vi "DecodeStreamResponse.vi"(0 "Buffer":string) -> (18 "ChecksumVerified":bool, 19 "Flags":u32, 20 "Gyroscope Full Scale Range":u32, 21 "Accelerometer Full Scale Range":u32, 22 "Output Rate":u32, 23 "Calibrated Yaw Offset":dbl, 24 "Calibrated Quaternion W Offset":u32, 25 "Calibrated Quaternion X Offset":u32, 26 "Calibrated Quaternion Y Offset":u32, 27 "Calibrated Quaternion Z Offset":u32)   [LabVIEW 2015, in "Nav6.lvlib"]
uses:
  Nav6.lvlib
panel:
  out "Stream Command Received":string
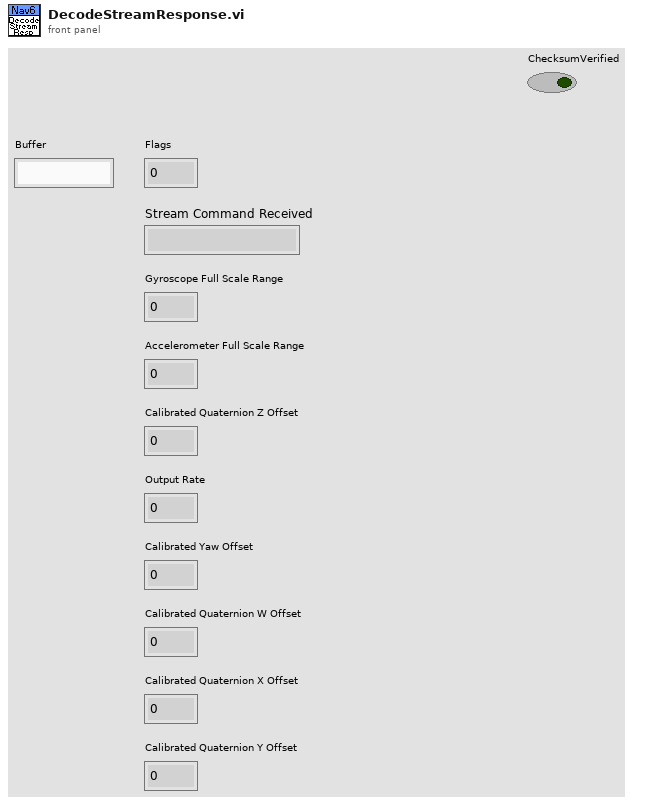
[diagram p1: front panel]
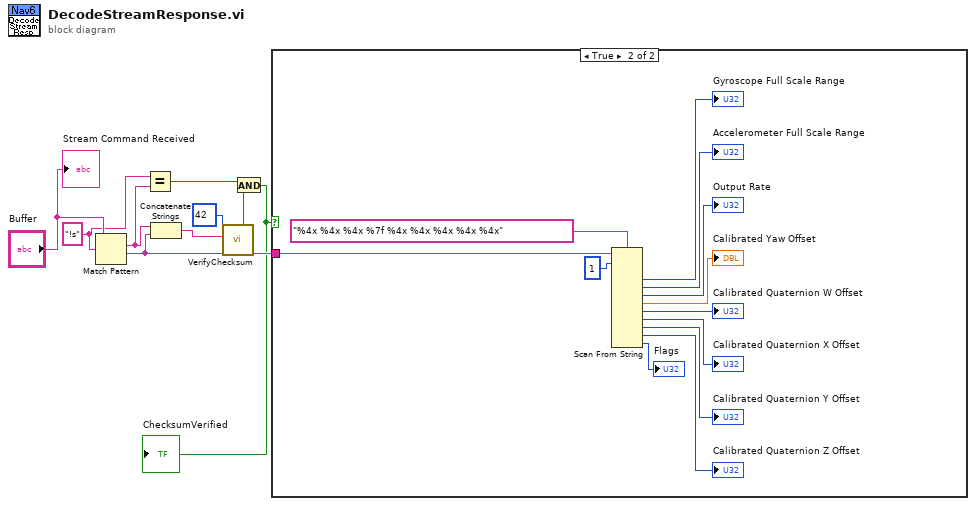
[diagram p0: block diagram]
diagram:
  w4 = "!s" ("string")
  n1 = Match Pattern(string="Buffer", regular expression=w4) -> (match substring=w5:string, after substring=w9:string)  [unwired: 1 in, 2 out]
  n2 = Equal?(x=w4, y=w5) -> (x = y?=w3:bool)
  n3 = Concatenate Strings(w5, w9) -> (w7:string)
  n4 = call "VerifyChecksum.vi"("String"=w7, "ChecksumIndex"=42) -> ("ChecksumVerified"=w2:bool)  [unwired: 9 in]
  n5 = And(x=w3, y=w2) -> (x .and. y?=w1:bool)
  "ChecksumVerified" <- w1
  n6 = case shown="True" w1 {
    tunnel: w9 -> [_ w21]
    frame False {
    }
    frame True {
      n7 = Scan From String(format string="%4x %4x %4x %7f %4x %4x %4x %4x %4x", input string=w21, initial scan location=u32 1) -> (output 1=→"Gyroscope Full Scale Range":u32, output 2=→"Accelerometer Full Scale Range":u32, output 3=→"Output Rate":u32, output 4=→"Calibrated Yaw Offset":dbl, output 5=→"Calibrated Quaternion W Offset":u32, output 6=→"Calibrated Quaternion X Offset":u32, output 7=→"Calibrated Quaternion Y Offset":u32, output 8=→"Calibrated Quaternion Z Offset":u32, output 9=→"Flags":u32)  [unwired: 10 in, 3 out]
    }
  }
  "Stream Command Received" <- "Buffer"
